vi "Valid_Message.vi"(6 "Max per day":i32, 8 "day of month in":i32, 9 "Number of requests today In":i32) -> (0 "day of month out":i32, 1 "Number of requests today Out":i32, 2 "Send Message":bool)   [LabVIEW 2010]
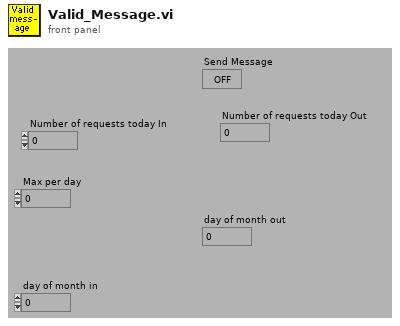
[diagram p1: front panel]
types:
  T1 = cluster{"second":i32, "minute":i32, "hour":i32, "day of month":i32, "month":i32, "year":i32, "day of week":i32, "day of year":i32, "is DST":i32}
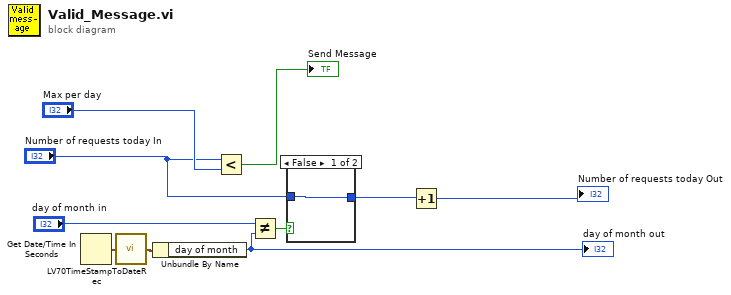
[diagram p0: block diagram]
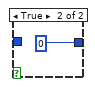
[diagram p2: hidden frame]
diagram:
  n1 = Get Date/Time In Seconds() -> (seconds since 1Jan1904=w1:timestamp)
  n2 = call <vilib>:"LV70TimeStampToDateRec.vi"("time stamp"=w1) -> ("date time rec"=w3:T1)
  n3 = Unbundle By Name(w3) -> ("day of month"=w5:i32)
  "day of month out" <- w5
  n4 = Less?(x="Number of requests today In", y="Max per day") -> (x < y?=→"Send Message":bool)
  n5 = Not Equal?(x="day of month in", y=w5) -> (x != y?=w6:bool)
  n6 = case shown="False" w6 {
    tunnel: "Number of requests today In" -> [w11 _]
    tunnel: [w11 0] -> w9
    frame False {
    }
    frame True {
    }
  }
  n7 = Increment(x=w9) -> (x+1=→"Number of requests today Out":i32)
